vi "CMN_toFits.vi"(4 "ms timeout (-1)":i32=-1, 5 "response Q":string, 6 "key":string, 7 "error in (no error)":errorcluster, 8 "data":u16[](array[numeric]), 9 "eleRead":u32[](array[numeric]), 10 "location":u64, 11 "command":string) -> (0 "error out":errorcluster, 1 "response":errorcluster)   [LabVIEW 2016]
panel:
  in  "cmd struct":T1
  out "Output Cluster":T2
  in  "image data":T3
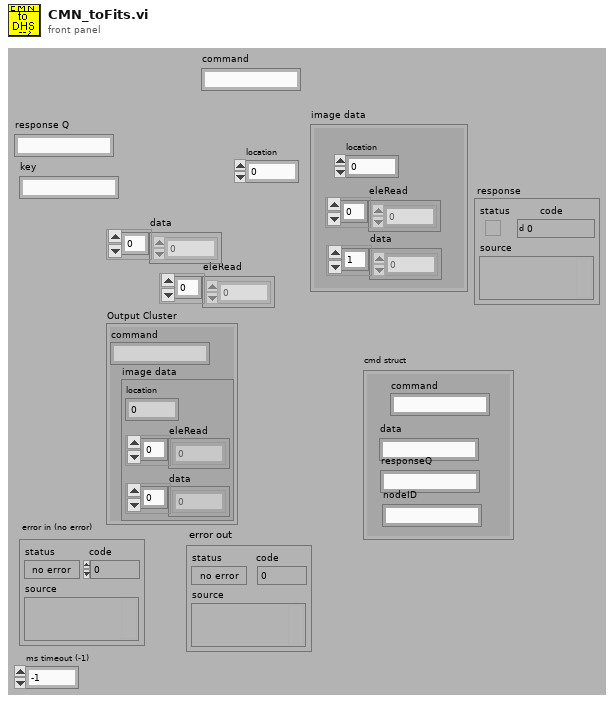
[diagram p1: front panel]
types:
  T1 = cluster{"command":string, "data":string, "responseQ":string, "nodeID":string}
  T2 = cluster{"command":string, "image data":cluster{"location":u32, "eleRead":u32[], "data":u16[]}}
  T3 = cluster{"location":u64, "eleRead":u32[], "data":u16[]}
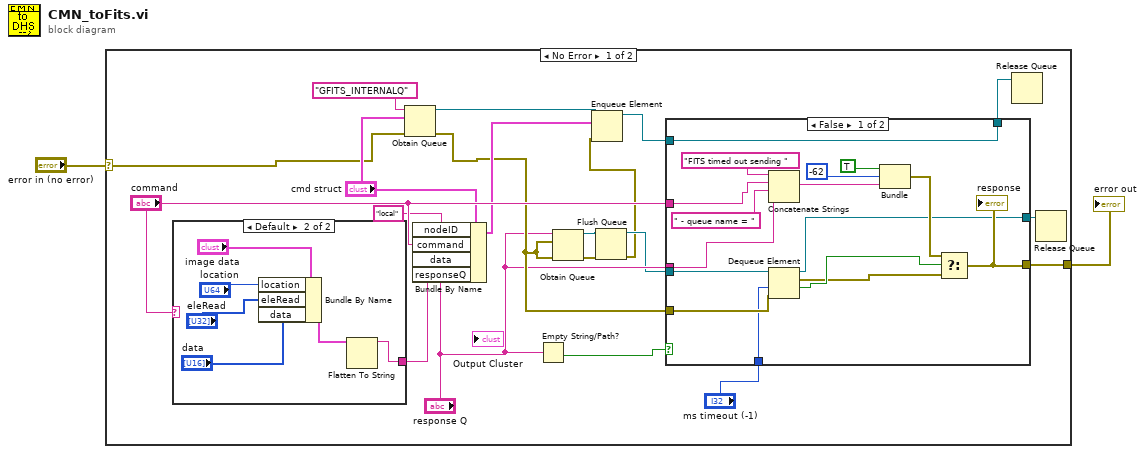
[diagram p0: block diagram]
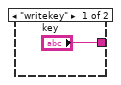
[diagram p3: hidden frame]
diagram:
  n1 = case shown="No Error" "error in (no error)" {
    selector: "error in (no error)" -> [w13 w49]
    tunnel: [w19 w49] -> w1
    frame No Error {
      n2 = case shown="Default" "command" {
        tunnel: ["key" w43] -> w22
        frame "writekey" {
        }
        frame Default {
          n3 = Bundle By Name(cluster="image data", "location"="location", "eleRead"="eleRead", "data"="data") -> (w44:T3)
          n4 = Flatten To String(anything=w44) -> (data string=w43:string)  [unwired: 1 in, 4 out]
        }
      }
      n5 = Obtain Queue(name (unnamed)="GFITS_INTERNALQ", element data type="cmd struct", error in (no error)=w13) -> (queue out=w16:refnum<queue>, error out=w9:errorcluster)  [unwired: 2 in, 1 out]
      n6 = Bundle By Name(cluster="cmd struct", "nodeID"="local", "command"="command", "data"=w22, "responseQ"="response Q") -> (w14:T1)
      n7 = Empty String/Path?(string/path="response Q") -> (empty?=w21:bool)
      n8 = Obtain Queue(name (unnamed)="response Q", element data type=w9, error in (no error)=w9) -> (queue out=w7:refnum<queue>, error out=w6:errorcluster)  [unwired: 2 in, 1 out]
      n9 = Flush Queue(queue=w7, error in (no error)=w6) -> (queue out=w5:refnum<queue>, error out=w4:errorcluster)  [unwired: 1 out]
      n10 = Enqueue Element(queue=w16, element=w14, error in (no error)=w4) -> (queue out=w12:refnum<queue>)  [unwired: 3 out]
      n11 = case shown="False" w21 {
        tunnel: "response Q" -> [w30 _]
        tunnel: "ms timeout (-1)" -> [w26 _]
        tunnel: w9 -> [w29 w41]
        tunnel: [w38 w41] -> w19
        tunnel: "command" -> [w37 _]
        tunnel: w12 -> [w25 w40]
        tunnel: [w25 w40] -> w11
        tunnel: [w24 w39] -> w10
        tunnel: w5 -> [w23 w39]
        frame False {
          n12 = Concatenate Strings("FITS timed out sending " ("source"), w37, " - queue name = ", w30) -> (w34:string)
          n13 = Dequeue Element(queue=w23, timeout in ms (-1)=w26, error in (no error)=w29) -> (queue out=w24:refnum<queue>, element=w27:errorcluster, timed out?=w28:bool)  [unwired: 1 out]
          n14 = Bundle(TRUE, -62, w34) -> (w35:errorcluster)  [unwired: 1 out]
          n15 = Select(t=w35, s=w28, f=w27) -> (s? t:f=w38:errorcluster)
          "response" <- w38
        }
        frame True {
        }
      }
      n16 = Release Queue(queue=w11) -> ()  [unwired: 1 in, 4 out]
      n17 = Release Queue(queue=w10) -> ()  [unwired: 1 in, 4 out]
    }
    frame Error {
    }
  }
  "error out" <- w1
